vi "Init.vi"(8 "error in":errorcluster, 11 "CFG Base in":refnum<class "Red-y Pressure Control CFG Simulated.lvclass">) -> (0 "error out":errorcluster, 3 "CFG Base out":refnum<class "Red-y Pressure Control CFG Simulated.lvclass">)   [LabVIEW 2024, in "Red-y Pressure Control CFG Simulated.lvclass"]
uses:
  Red-y Pressure Control CFG Simulated.lvclass
  Configurations/CFG Base/CFG Base.lvclass/CFG Base.ctl
  Pressure Control CFG/Red-y Pressure Control CFG.lvclass
  Configurations/CFG Base/CFG Base.lvclass
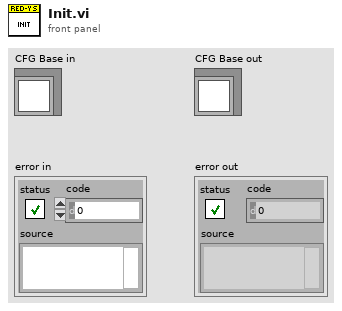
[diagram p1: front panel]
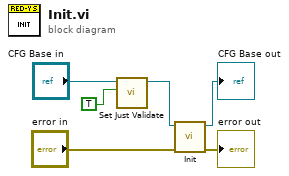
[diagram p0: block diagram]
diagram:
  n1 = call "Set Just Validate.vi"("Just Validate"=TRUE, "CFG Base in"="CFG Base in") -> ("CFG Base out"=w2:refnum<class "Red-y Pressure Control CFG Simulated.lvclass">)  [unwired: 9 in]
  n2 = call-parent "Init.vi"("error in"="error in", "CFG Base in"=w2) -> ("error out"=→"error out":errorcluster, "CFG Base out"=→"CFG Base out":refnum<class "Red-y Pressure Control CFG Simulated.lvclass">)  [unwired: 8 in]
